vi "SetTdmsFileOut.vi"(0 "object in":refnum<class "TDMSLogger_PowerScan.lvclass">, 1 "tdms file out":refnum<k34>, 5 "error in (no error)":errorcluster) -> (14 "object out":refnum<class "TDMSLogger_PowerScan.lvclass">, 19 "error out":errorcluster)   [LabVIEW 2023, in "TDMSLogger_PowerScan.lvclass"]
uses:
  TDMSLogger_PowerScan.lvclass
  TDMSLogger_PowerScan.lvclass/TDMSLogger_PowerScan.ctl
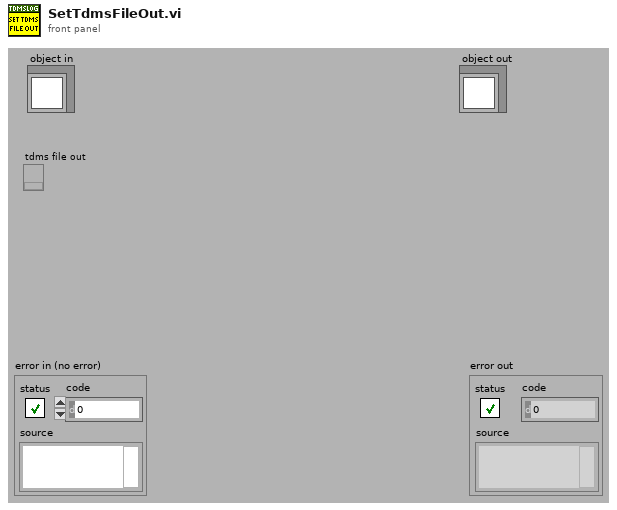
[diagram p1: front panel]
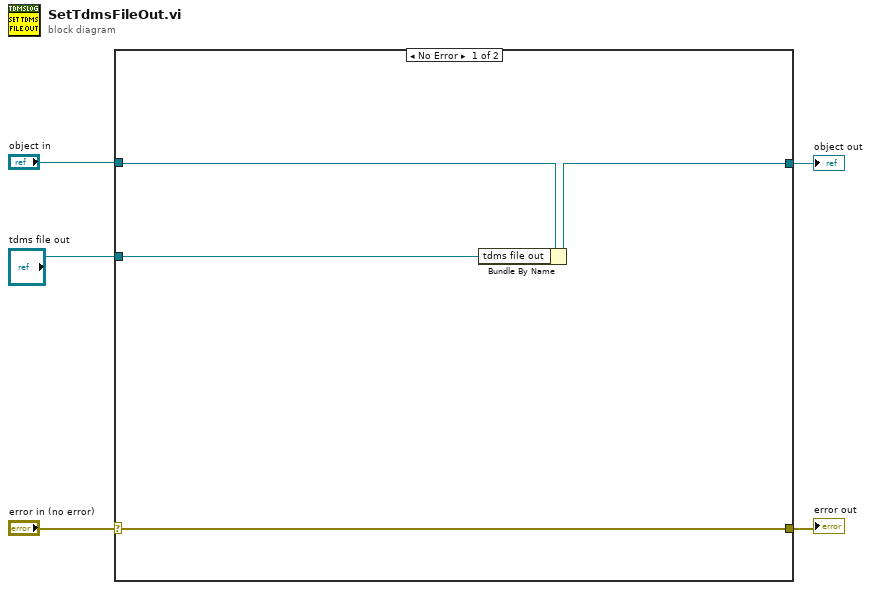
[diagram p0: block diagram]
diagram:
  n1 = case shown="No Error" "error in (no error)" {
    selector: "error in (no error)" -> [w8 w11]
    tunnel: [w8 w11] -> w4
    tunnel: [w6 w10] -> w2
    tunnel: "object in" -> [w7 w10]
    tunnel: "tdms file out" -> [w9 _]
    frame No Error {
      n2 = Bundle By Name(cluster=w7, "tdms file out"=w9) -> (w6:refnum<class "TDMSLogger_PowerScan.lvclass">)
    }
    frame Error {
    }
  }
  "error out" <- w4
  "object out" <- w2
